vi "Write Channel Current Limint.vi"(10 "Channel Current Limit":dbl[](array[numeric]), 11 "E3631A in":refnum<class "E3631A.lvclass">) -> (3 "E3631A out":refnum<class "E3631A.lvclass">)   [LabVIEW 2020, in "E3631A.lvclass"]
uses:
  E3631A.lvclass
  E3631A.lvclass/E3631A.ctl
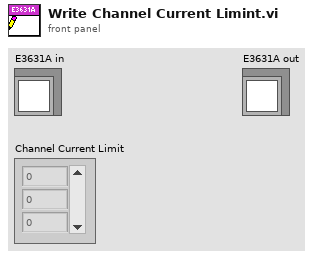
[diagram p1: front panel]
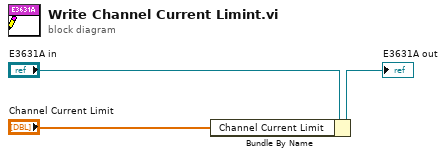
[diagram p0: block diagram]
diagram:
  n1 = Bundle By Name(cluster="E3631A in", "Channel Current Limit"="Channel Current Limit") -> (→"E3631A out":refnum<class "E3631A.lvclass">)
